vi "Configurações de Usuário.vi"() -> ()   [LabVIEW 2020]
uses:
  <vilib>/Utility/file.llb/Read Delimited Spreadsheet (string).vi
  <vilib>/Utility/file.llb/Write Delimited Spreadsheet (string).vi
panel:
  in  "Turno de trabalho":string(combo)
  in  "Nível de permissões":string(combo)
  in  "Função":string(combo)
  in  "ID":u8
  in  "Salvar":bool
  in  "Add Novo Usuário":bool
  in  "Usuário":string(combo)
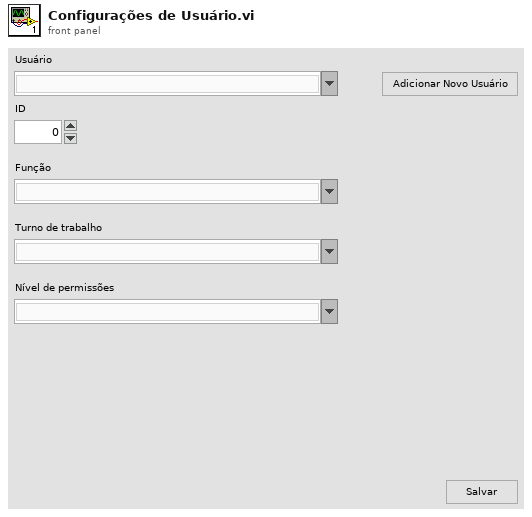
[diagram p1: front panel]
types:
  T1 = typedef "Estados da configuração de usuário.ctl" = enum16{"Inicializar", "Aguardar Evento", "Salvar", "Atualizar infos da Tela", "Novo usuário"}
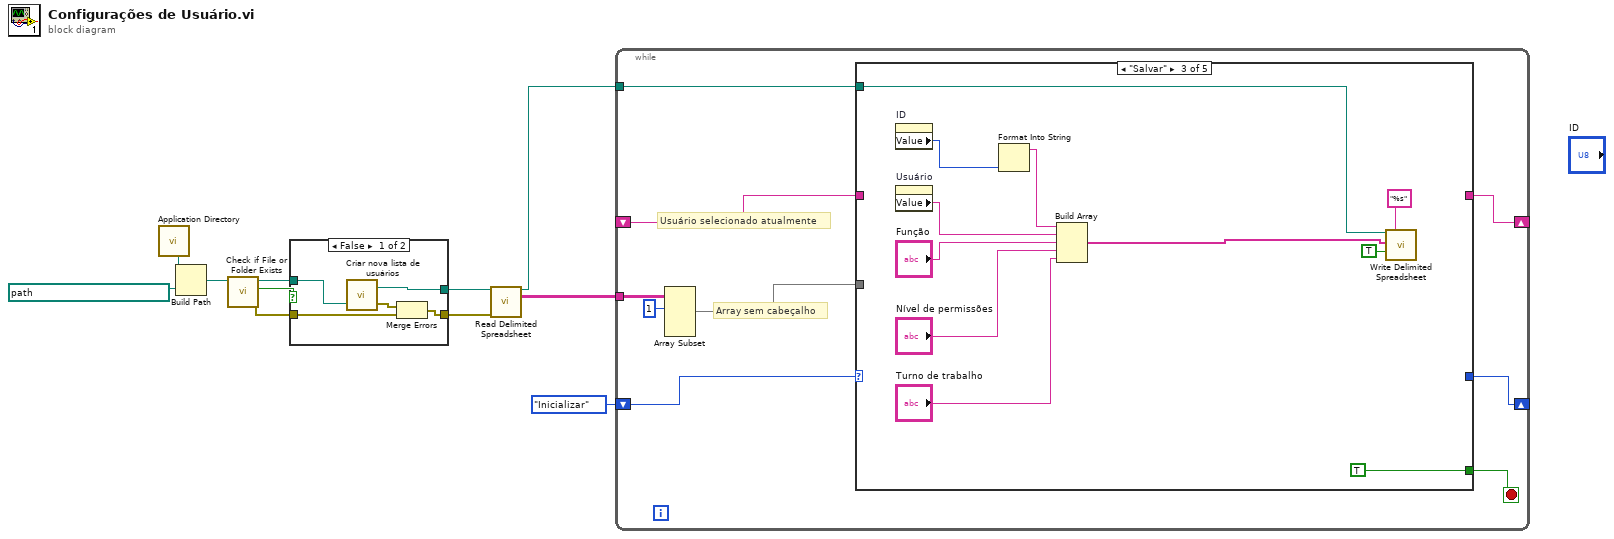
[diagram p0: block diagram]
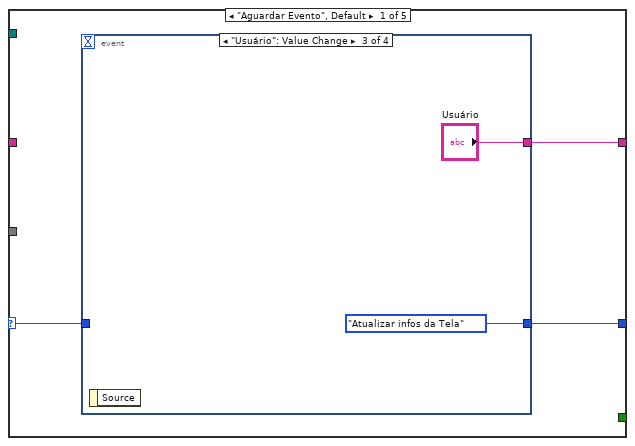
[diagram p3: hidden frame]
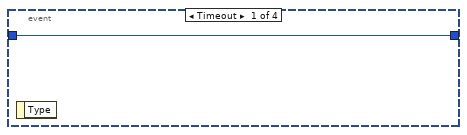
[diagram p4: hidden frame]
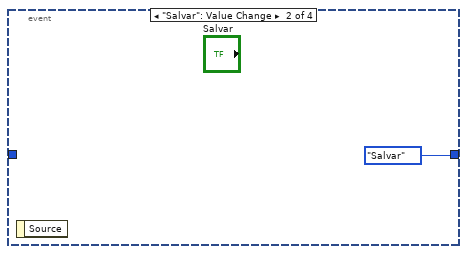
[diagram p5: hidden frame]
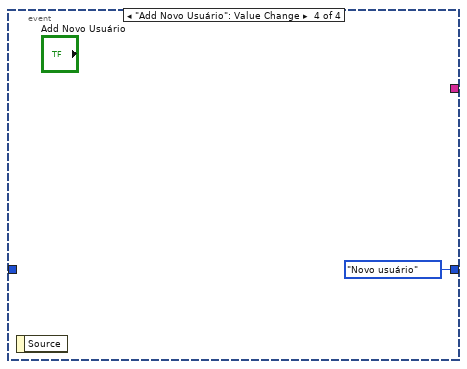
[diagram p6: hidden frame]
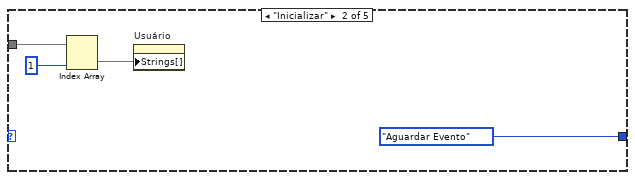
[diagram p7: hidden frame]
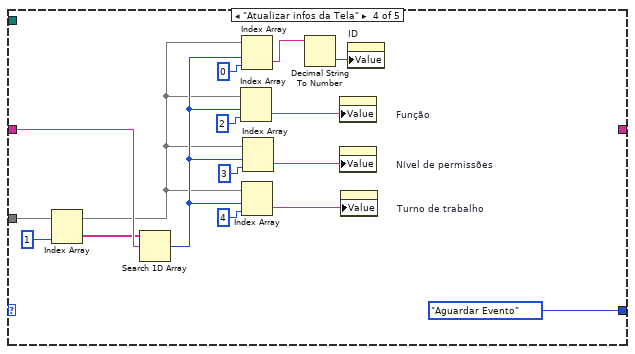
[diagram p8: hidden frame]
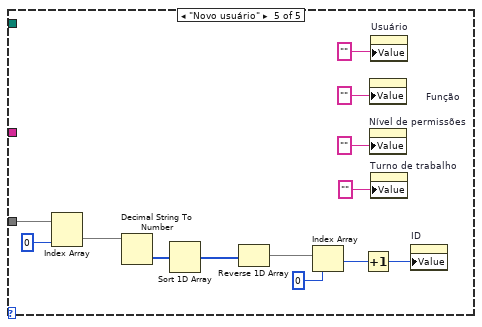
[diagram p9: hidden frame]
diagram:
  n1 = call <vilib>:"Application Directory.vi"() -> ("Application Directory"=w10:path)
  n2 = Build Path(base path=w10, name or relative path=path "Configurações/Usuários.csv") -> (appended path=w11:path)
  n3 = call <vilib>:"Check if File or Folder Exists.vi"("path"=w11) -> ("error out"=w6:errorcluster, "file or folder exists?"=w8:bool, "dup path"=w7:path)  [unwired: 8 in]
  n4 = case shown="False" w8 {
    tunnel: w7 -> [w16 w18]
    tunnel: w6 -> [w14 w17]
    tunnel: [w13 w18] -> w5
    tunnel: [w12 w17] -> w4
    frame False {
      n5 = call "Criar nova lista de usuários.vi"("Path"=w16) -> ("error out"=w15:errorcluster, "file path"=w13:path)  [unwired: 1 in]
      n6 = Merge Errors(w15, w14) -> (w12:errorcluster)
    }
    frame True {
    }
  }
  n7 = call-poly <vilib>:"Read Delimited Spreadsheet.vi"("file path (dialog if empty)"=w5, "error in (no error)"=w4) -> ("new file path (Not A Path if cancelled)"=w1:path, "all rows"=w3:string[][])  [unwired: 8 in, 4 out]
  n8 = while {
    shift-right: [w27] -> _
    shift-left: Estados_da_configuração_de_usuário."Inicializar" -> [w26]
    tunnel: w3 -> [w20]
    shift-right: [w24] -> _
    shift-left: _ -> [w23]
    tunnel: w1 -> [w19]
    stop <- w25 stop-if-true
    # "Usuário selecionado atualmente"
    # "Array sem cabeçalho"
    n9 = Array Subset(array=w20, index (row)=1 ("index")) -> (w21:string[][])  [unwired: 3 in]
    n10 = case shown="\"Salvar\"" w26 {
      selector: w26 -> [w29 _ _ _ _]
      tunnel: [w30 Estados_da_configuração_de_usuário."Aguardar Evento" _ Estados_da_configuração_de_usuário."Aguardar Evento" _] -> w27
      tunnel: [_ _ TRUE _ _] -> w25
      tunnel: [w28 _ _ _ _] -> w24
      tunnel: w23 -> [_ _ _ w64 _]
      tunnel: w21 -> [_ w36 _ w53 w74]
      tunnel: w19 -> [_ _ w43 _ _]
      frame "Aguardar Evento", Default {
        n11 = event shown="[2] \"Usuário\": Value Change" {
          selector: _ -> [_ _ _ _]
          dyn-events: _ -> [_ _ _ _]
          timeout: _ -> [_ _ _ _]
          tunnel: [w31 Estados_da_configuração_de_usuário."Salvar" Estados_da_configuração_de_usuário."Atualizar infos da Tela" Estados_da_configuração_de_usuário."Novo usuário"] -> w30
          tunnel: w29 -> [w31 _ _ _]
          tunnel: [_ _ "Usuário" _] -> w28
          event Timeout {
            n12 = event-data() -> ()  [unwired: 1 in, 1 out]
          }
          event "Salvar": Value Change {
            n13 = event-data() -> ()  [unwired: 1 in, 1 out]
          }
          event "Usuário": Value Change {
            n14 = event-data() -> ()  [unwired: 1 in, 1 out]
          }
          event "Add Novo Usuário": Value Change {
            n15 = event-data() -> ()  [unwired: 1 in, 1 out]
          }
        }
      }
      frame "Inicializar" {
        n16 = Index Array(array=w36, index (col)=1 ("disabled index (col)")) -> (element=w39:string[])  [unwired: 1 in]
        n17 = property on="Usuário" class="CmbBox"("Strings[]"=w39) -> ()  [unwired: 2 in, 2 out]
      }
      frame "Salvar" {
        n18 = property on="ID" class="DigNum (strict)"() -> ("Value"=w48:u8)  [unwired: 2 in, 2 out]
        n19 = property on="Usuário" class="CmbBox"() -> ("Value"=w49:string)  [unwired: 2 in, 2 out]
        n20 = Format Into String(w48) -> (resulting string=w47:string)  [unwired: 3 in, 1 out]
        n21 = Build Array(w47, w49, "Função", "Nível de permissões", "Turno de trabalho") -> (w40:string[])
        n22 = call-poly <vilib>:"Write Delimited Spreadsheet.vi"("file path (dialog if empty)"=w43, "format (%s)"="%s", "1D data"=w40, "append to file? (new file:F)"=TRUE) -> ()  [unwired: 10 in, 2 out]
      }
      frame "Atualizar infos da Tela" {
        n23 = Index Array(array=w53, index (col)=1 ("disabled index (col)")) -> (element=w63:string[])  [unwired: 1 in]
        n24 = Search 1D Array(1D array=w63, element=w64) -> (index of element=w55:i32)  [unwired: 1 in]
        n25 = Index Array(array=w53, index (row)=w55, index (col)=2 ("disabled index (col)")) -> (element=w59:string)
        n26 = Index Array(array=w53, index (row)=w55, index (col)=0 ("disabled index (col)")) -> (element=w52:string)
        n27 = Index Array(array=w53, index (row)=w55, index (col)=4 ("disabled index (col)")) -> (element=w54:string)
        n28 = Index Array(array=w53, index (row)=w55, index (col)=3 ("disabled index (col)")) -> (element=w58:string)
        n29 = Decimal String To Number(string=w52) -> (number=w51:i32)  [unwired: 2 in, 1 out]
        n30 = property on="Função" class="CmbBox"("Value"=w59) -> ()  [unwired: 2 in, 2 out]
        n31 = property on="Nível de permissões" class="CmbBox"("Value"=w58) -> ()  [unwired: 2 in, 2 out]
        n32 = property on="Turno de trabalho" class="CmbBox"("Value"=w54) -> ()  [unwired: 2 in, 2 out]
        n33 = property on="ID" class="DigNum (strict)"("Value"=w51) -> ()  [unwired: 2 in, 2 out]
      }
      frame "Novo usuário" {
        n34 = Index Array(array=w74, index (col)=0 ("disabled index (col)")) -> (element=w73:string[])  [unwired: 1 in]
        n35 = Decimal String To Number(string=w73) -> (number=w72:i32[])  [unwired: 2 in, 1 out]
        n36 = Sort 1D Array(array=w72) -> (sorted array=w68:i32[])
        n37 = Reverse 1D Array(array=w68) -> (reversed array=w67:i32[])
        n38 = Index Array(array=w67, index=0) -> (element=w70:i32)
        n39 = Increment(x=w70) -> (x+1=w69:i32)
        n40 = property on="Função" class="CmbBox"("Value"="" ("Text.Text")) -> ()  [unwired: 2 in, 2 out]
        n41 = property on="Nível de permissões" class="CmbBox"("Value"="" ("Text.Text")) -> ()  [unwired: 2 in, 2 out]
        n42 = property on="Usuário" class="CmbBox"("Value"="") -> ()  [unwired: 2 in, 2 out]
        n43 = property on="Turno de trabalho" class="CmbBox"("Value"="" ("Text.Text")) -> ()  [unwired: 2 in, 2 out]
        n44 = property on="ID" class="DigNum (strict)"("Value"=w69) -> ()  [unwired: 2 in, 2 out]
      }
    }
  }
